vi "LightSensorStart.vi"(0 "Device Info":T1={"Serial Number"=-1, "Channel"=0, "Port"=0}, 1 "Data Interval":i32=-1, 2 "Change Trigger":dbl, 11 "error in (no error)":errorcluster, 12 "Connection":u16(ring) items=["No Preference", "Remote", "Local"], 13 "Timeout (mSec)":i32=5000) -> (4 "Phidget ID":u64, 6 "Serial Number Return":i32, 10 "Attached?":bool, 15 "error out":errorcluster)   [LabVIEW 2012, in "Phidget Light Sensor.lvlib"]
doc: "${LightSensor:StartHeader}"
uses:
  <instrlib>/Phidgets/Phidget Light Sensor/Phidget Light Sensor.lvlib
  <instrlib>/Phidgets/Phidget Common/Phidget Common.lvlib
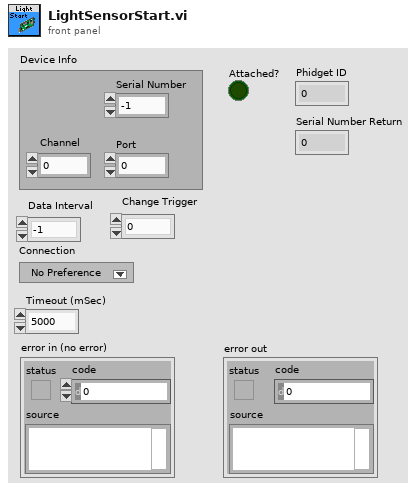
[diagram p1: front panel]
types:
  T1 = cluster{"Serial Number":i32, "Channel":i32, "Port":i32}
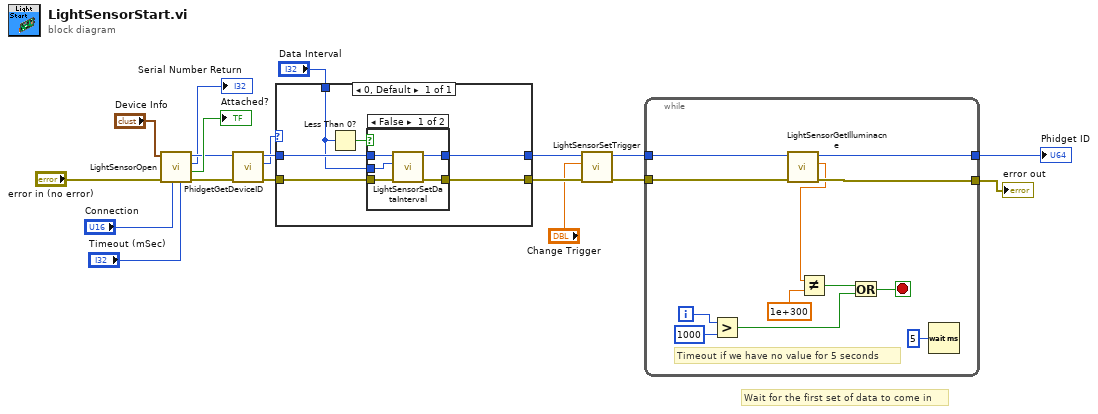
[diagram p0: block diagram]
diagram:
  # "Wait for the first set of data to come in"
  n1 = call <instrlib>:"LightSensorOpen.vi"("Timeout (mSec)"="Timeout (mSec)", "Connection"="Connection", "error in"="error in (no error)", "Device Info"="Device Info") -> ("error out"=w16:errorcluster, "Attached?"=→"Attached?":bool, "Serial Number Return"=→"Serial Number Return":i32, "Phidget ID"=w15:u64)  [unwired: 4 in]
  n2 = call <instrlib>:"PhidgetGetDeviceID.vi"("error in (no error)"=w16, "Device In"=w15) -> ("error out"=w13:errorcluster, "Devie IDs"=w12:u32, "Device Out"=w14:u64)  [unwired: 6 in]
  n3 = case shown="0, Default" w12 {
    tunnel: w13 -> [w24]
    tunnel: [w20] -> w6
    tunnel: w14 -> [w23]
    tunnel: [w21] -> w7
    tunnel: "Data Interval" -> [w22]
    frame 0, Default {
      n4 = Less Than 0?(x=w22) -> (x < 0?=w25:bool)
      n5 = case shown="False" w25 {
        tunnel: w23 -> [w30 w32]
        tunnel: w24 -> [w29 w31]
        tunnel: [w27 w32] -> w21
        tunnel: [w28 w31] -> w20
        tunnel: w22 -> [w26 _]
        frame False {
          n6 = call <instrlib>:"LightSensorSetDataInterval.vi"("error in (no error)"=w29, "Interval"=w26, "Device In"=w30) -> ("error out"=w28:errorcluster, "Device Out"=w27:u64)  [unwired: 6 in]
        }
        frame True {
        }
      }
    }
  }
  n7 = call <instrlib>:"LightSensorSetTrigger.vi"("error in (no error)"=w6, "Trigger"="Change Trigger", "Device In"=w7) -> ("error out"=w8:errorcluster, "Device Out"=w9:u64)  [unwired: 6 in]
  n8 = while {
    tunnel: w9 -> [w42]
    tunnel: w8 -> [w41]
    tunnel: [w39] -> w11
    tunnel: [w40] -> w18
    i -> [w37]
    stop <- w34 stop-if-true
    # "Timeout if we have no value for 5 seconds"
    n9 = Greater?(x=w37, y=1000) -> (0:w35:bool)
    n10 = call <instrlib>:"LightSensorGetIlluminacne.vi"("error in (no error)"=w41, "Device In"=w42) -> ("error out"=w40:errorcluster, "Illuminance"=w33:dbl, "Device Out"=w39:u64)  [unwired: 6 in]
    n11 = Not Equal?(x=w33, y=1e+300) -> (x != y?=w36:bool)
    n12 = Or(x=w36, y=w35) -> (x .or. y?=w34:bool)
    n13 = Wait (ms)(milliseconds to wait=u32 5) -> ()  [unwired: 1 out]
  }
  "error out" <- w18
  "Phidget ID" <- w11
